vi "Prober_ThetaAlignment.vi"(4 "y2":i32, 5 "y1":i32, 6 "x2":i32, 7 "x1":i32, 8 "error in (no error)":errorcluster, 11 "AlessiRel6100 in":refnum<class "AlessiRel6100.lvclass">) -> (0 "error out":errorcluster, 1 "theta increment":i32, 2 "New millidegrees":i32, 3 "AlessiRel6100 out":refnum<class "AlessiRel6100.lvclass">)   [LabVIEW 2018, in "AlessiRel6100.lvclass"]
uses:
  AlessiRel6100.lvclass
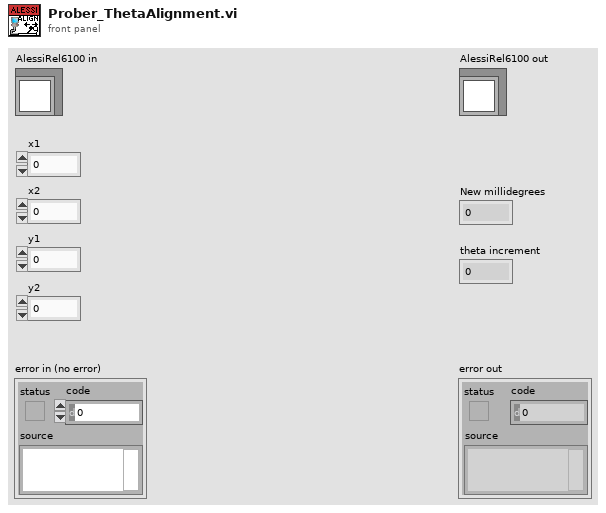
[diagram p1: front panel]
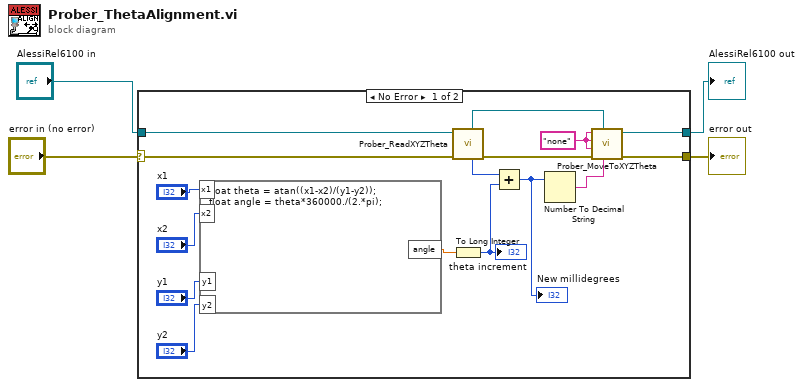
[diagram p0: block diagram]
diagram:
  n1 = case shown="No Error" "error in (no error)" {
    selector: "error in (no error)" -> [w15 w21]
    tunnel: "AlessiRel6100 in" -> [w20 w22]
    tunnel: [w18 w22] -> w2
    tunnel: [w17 w21] -> w1
    frame No Error {
      w14 = "none"
      n2 = formula code="float theta = atan((x1-x2)/(y1-y2));\nfloat angle = theta*360000./(2.*pi);"("x1"="x1", "x2"="x2", "y1"="y1", "y2"="y2") -> ("angle"=w8:dbl)
      n3 = call-dynamic "Prober_ReadXYZTheta.vi"("error in (no error)"=w15, "AlessiRel6100 in"=w20) -> ("error out"=w16:errorcluster, "Theta location [mdeg]"=w9:i32, "AlessiRel6100 out"=w19:refnum<class "AlessiRel6100.lvclass">)  [unwired: 4 in, 3 out]
      n4 = To Long Integer(number=w8) -> (32bit integer=w7:i32)
      "theta increment" <- w7
      n5 = Add(x=w9, y=w7) -> (x+y=w6:i32)
      "New millidegrees" <- w6
      n6 = Number To Decimal String(number=w6) -> (decimal integer string=w5:string)  [unwired: 1 in]
      n7 = call-dynamic "Prober_MoveToXYZTheta.vi"("Theta location [mdeg]"=w5, "AlessiRel6100 in"=w19, "error in (no error)"=w16, "Z location [µm]"=w14, "Y location [µm]"=w14, "X location [µm]"=w14) -> ("error out"=w17:errorcluster, "AlessiRel6100 out"=w18:refnum<class "AlessiRel6100.lvclass">)  [unwired: 3 in, 1 out]
    }
    frame Error {
    }
  }
  "error out" <- w1
  "AlessiRel6100 out" <- w2
